vi "PIMAX_1.vi"() -> ()   [LabVIEW 2018]
uses:
  <vilib>/Enthought/Python Integration Toolkit/api/Console Visibility.ctl
  Global Variables.vi
  <vilib>/Enthought/Python Integration Toolkit/Python Integration Toolkit.lvlib
panel:
  in  "Experiment Name":string="TestCamera"
  in  "Logfile?":bool
  in  "File Path":path=path "C:/Labview Test Data/2018-10-09/UnspecifiedProj/Temp Dependence/PIMAX_1_500C_9"
  in  "stop":bool
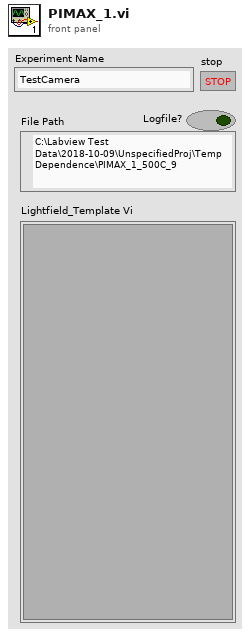
[diagram p1: front panel]
types:
  T1 = typedef "Python Integration Toolkit.lvlib/Console Visibility.ctl" = enum16{"Show Console", "Show Console While Running", "Hide Console"}
  T2 = enum32{"Bad", "Idle", "Run top level", "Running"}
  T3 = typedef "Python Integration Toolkit.lvlib/Session ID.ctl" = u64
  T4 = cluster{"Project":u16, "SubFolder":string, "Filename (Meas. Description)":string, "Measurement index":i32}
  T5 = typedef "Python Integration Toolkit.lvlib/Python Objects.ctl" = variant
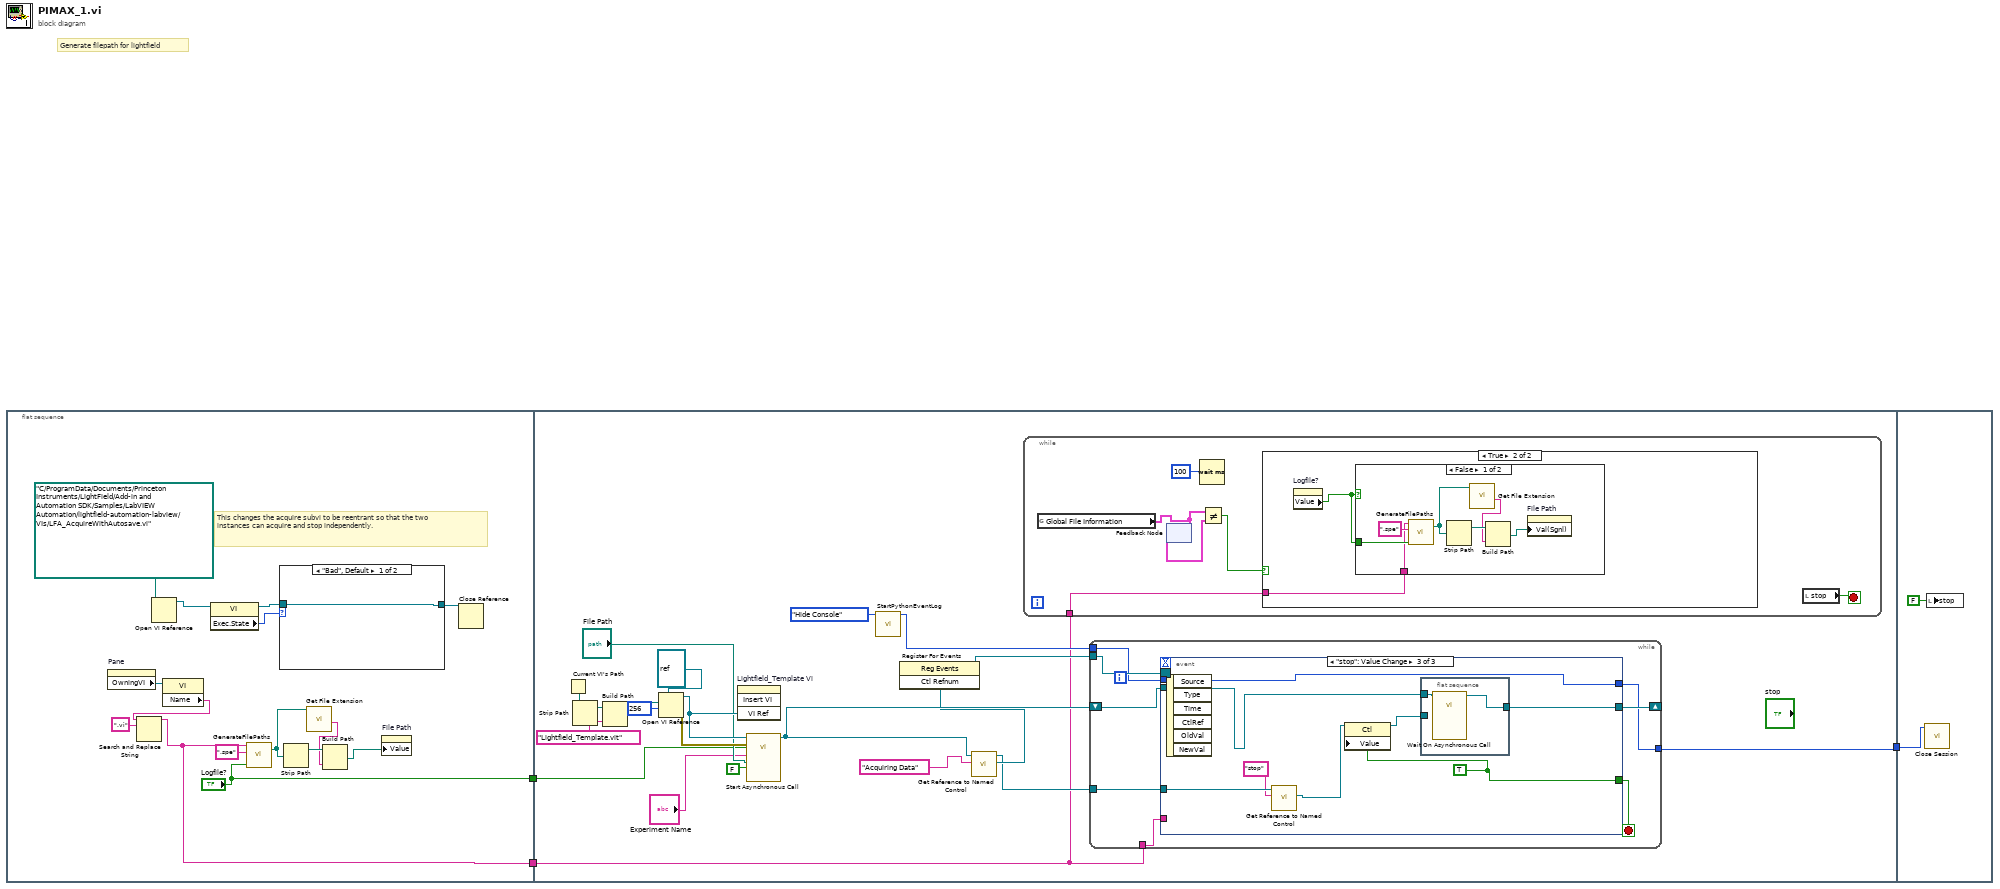
[diagram p0: block diagram]
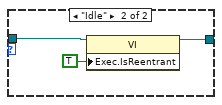
[diagram p2: hidden frame]
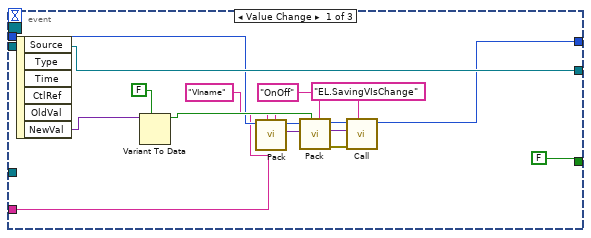
[diagram p5: hidden frame]
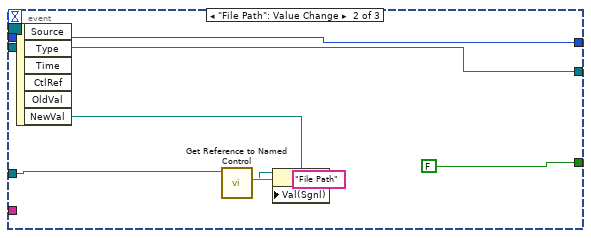
[diagram p6: hidden frame]
diagram:
  # "Generate filepath for lightfield"
  n1 = flat-sequence {
    tunnel: [w5] -> w2
    tunnel: ["Logfile?"] -> w1
    tunnel: [w32] -> w3
    tunnel: w2 -> [w25]
    tunnel: w1 -> [w24]
    tunnel: w3 -> [w100]
    frame #0 {
      # "This changes the acquire subvi to be reentrant so that the two instances can acquire and stop independently."
      n2 = property on="Pane" class="Pane"() -> ("OwningVI"=w8:refnum<vi>)  [unwired: 2 in, 2 out]
      n3 = Open VI Reference(vi path=path "C:/ProgramData/Documents/Princeton Instruments/LightField/Add-in and Automation SDK/Samples/LabVIEW Automation/lightfield-automation-labview/VIs/LFA_AcquireWithAutosave.vi") -> (vi reference=w11:refnum<vi>)  [unwired: 5 in, 1 out]
      n4 = property class="VI"(reference=w8) -> ("Name"=w6:string)  [unwired: 1 in, 2 out]
      n5 = Search and Replace String(input string=w6, search string=".vi") -> (result string=w5:string)  [unwired: 6 in, 3 out]
      n6 = property class="VI"(reference=w11) -> (reference out=w9:refnum<vi>, "Exec.State"=w10:T2)  [unwired: 1 in, 1 out]
      n7 = call "GenerateFilePaths.vi"("Logfile? (F)"="Logfile?", "Extension (.tdms)"=".spe" ("Extension"), "Device Name"=w5) -> ("Path"=w15:path)  [unwired: 2 in]
      n8 = case shown="\"Bad\", Default" w10 {
        tunnel: [w19 w21] -> w17
        tunnel: w9 -> [w19 w20]
        frame "Bad", Default {
        }
        frame "Idle" {
          n9 = property class="VI"(reference=w20, "Exec.IsReentrant"=TRUE ("Execution:Is Reentrant")) -> (reference out=w21:refnum<vi>)  [unwired: 1 in, 1 out]
        }
      }
      n10 = Strip Path(path=w15) -> (stripped path=w14:path)  [unwired: 1 out]
      n11 = call <vilib>:"Get File Extension.vi"("file"=w15) -> ("filename without extension"=w13:string)  [unwired: 6 in, 4 out]
      n12 = Build Path(base path=w14, name or relative path=w13) -> (appended path=w12:path)
      n13 = property on="File Path" class="Path"("Value"=w12) -> ()  [unwired: 2 in, 2 out]
      n14 = Close Reference(reference=w17) -> ()  [unwired: 1 in, 1 out]
    }
    frame #1 {
      n15 = Current VI's Path() -> (path=w42:path)
      n16 = Strip Path(path=w42) -> (stripped path=w43:path)  [unwired: 1 out]
      n17 = Build Path(base path=w43, name or relative path="Lightfield_Template.vit") -> (appended path=w39:path)
      n18 = Open VI Reference(type specifier VI Refnum (for type only)=refnum<vi> refnum, vi path=w39, options=256) -> (vi reference=w38:refnum<vi>, error out=w37:errorcluster)  [unwired: 1 in, 2 out]
      n19 = invoke on="Lightfield_Template Vi" class="SubPnl" method="Insert VI"("VI Ref"=w38) -> ()  [unwired: 3 in, 4 out]
      n20 = call-by-ref "Start Asynchronous Call"(reference=w38, error in=w37, "Add Time to filename"=w24, "Single Run"=FALSE, "File Path"="File Path", "Experiment Name"="Experiment Name") -> (reference out=w31:refnum<vi>)  [unwired: 8 in, 1 out]
      n21 = call "StartPythonEventLog.vi"("Console Visibility"=Console_Visibility."Hide Console") -> ("Session ID out"=w33:T3)  [unwired: 10 in]
      n22 = call "Get Reference to Named Control.vi"("Control Name"="Acquiring Data" ("element"), "Front Panel Ref"=w31) -> ("Ctl Refnum"=w29:refnum<vi>, "Panel Ref Out"=w28:refnum<vi>)  [unwired: 7 in, 1 out]
      n23 = register-events(w29) -> (reference out=w34:refnum<event-registration>)  [unwired: 2 in, 1 out]
      n24 = while {
        tunnel: w25 -> [w44]
        stop <- w49 stop-if-true
        n25 = global read "Global Variables.vi" "Global File Information"() -> (w47:T4)
        n26 = feedback #1() -> (w46:T4)  [unwired: 1 in]
        n27 = feedback-in #1(w47) -> ()
        n28 = Wait (ms)(milliseconds to wait=100) -> ()  [unwired: 1 out]
        n29 = Not Equal?(x=w47, y=w46) -> (x != y?=w45:bool)
        n30 = case shown="True" w45 {
          tunnel: w44 -> [_ w50]
          frame False {
          }
          frame True {
            n31 = property on="Logfile?" class="Bool (strict)"() -> ("Value"=w51:bool)  [unwired: 2 in, 2 out]
            n32 = case shown="False" w51 {
              tunnel: w51 -> [w54 _]
              tunnel: w50 -> [w52 _]
              frame False {
                n33 = call "GenerateFilePaths.vi"("Logfile? (F)"=w54, "Extension (.tdms)"=".spe" ("Extension"), "Device Name"=w52) -> ("Path"=w57:path)  [unwired: 2 in]
                n34 = Strip Path(path=w57) -> (stripped path=w56:path)  [unwired: 1 out]
                n35 = call <vilib>:"Get File Extension.vi"("file"=w57) -> ("filename without extension"=w55:string)  [unwired: 6 in, 4 out]
                n36 = Build Path(base path=w56, name or relative path=w55) -> (appended path=w53:path)
                n37 = property on="File Path" class="Path"("Val(Sgnl)"=w53) -> ()  [unwired: 2 in, 2 out]
              }
              frame True {
              }
            }
          }
        }
        n38 = local read "stop"() -> (w49:bool)
      }
      n39 = while {
        shift-right: [w64] -> _
        shift-left: w31 -> [w65]
        tunnel: w34 -> [w63]
        tunnel: w33 -> [w62]
        tunnel: [w61] -> w32
        tunnel: w28 -> [w60]
        tunnel: w25 -> [w59]
        stop <- w66 stop-if-true
        n40 = event shown="[2] \"stop\": Value Change" {
          selector: w63 -> [_ _ _]
          dyn-events: _ -> [_ _ _]
          timeout: _ -> [_ _ _]
          tunnel: [FALSE FALSE w97] -> w66
          tunnel: w65 -> [w81 w87 w96]
          tunnel: [w81 w87 w95] -> w64
          tunnel: w62 -> [w75 w83 w90]
          tunnel: [w68 w83 w90] -> w61
          tunnel: w60 -> [_ w85 w93]
          tunnel: w59 -> [w67 _ _]
          event Value Change {
            n41 = event-data() -> ("NewVal"=w80:variant)  [unwired: 1 in, 5 out]
            n42 = Variant To Data(type=FALSE, Variant=w80) -> (data=w78:bool)  [unwired: 1 in, 1 out]
            n43 = call <vilib>:"Pack.vi"("Keyword Name"="VIname", "Argument"=w67, "Session ID"=w75) -> ("Python Object References Out"=w70:T5, "Session ID out"=w74:T3)  [unwired: 6 in, 1 out]
            n44 = call <vilib>:"Pack.vi"("Keyword Name"="OnOff", "Argument"=w78, "Python Object References In"=w70, "Session ID"=w74) -> ("error out"=w73:errorcluster, "Python Object References Out"=w72:T5, "Session ID out"=w71:T3)  [unwired: 5 in]
            n45 = call <vilib>:"Call.vi"("Function or Method Name"="EL.SavingVIsChange", "error in (no error)"=w73, "Python Object References In"=w72, "Session ID"=w71) -> ("Session ID out"=w68:T3)  [unwired: 5 in, 2 out]
          }
          event "File Path": Value Change {
            n46 = event-data() -> ("NewVal"=w89:path)  [unwired: 1 in, 5 out]
            n47 = call "Get Reference to Named Control.vi"("Control Name"="File Path" ("element"), "Front Panel Ref"=w85) -> ("Ctl Refnum"=w84:refnum<vi>)  [unwired: 7 in, 2 out]
            n48 = property class="Ctl"(reference=w84, "Val(Sgnl)"=w89) -> ()  [unwired: 1 in, 2 out]
          }
          event "stop": Value Change {
            w97 = TRUE
            n49 = event-data() -> ()  [unwired: 1 in, 6 out]
            n50 = call "Get Reference to Named Control.vi"("Control Name"="stop", "Front Panel Ref"=w93) -> ("Ctl Refnum"=w91:refnum<vi>)  [unwired: 7 in, 2 out]
            n51 = property class="Ctl"(reference=w91, "Value"=w97) -> (reference out=w94:refnum<vi>)  [unwired: 1 in, 1 out]
            n52 = flat-sequence {
              tunnel: w96 -> [w99]
              tunnel: w94 -> [_]
              tunnel: [w98] -> w95
              frame #0 {
                n53 = call-by-ref "Wait On Asynchronous Call"(reference=w99) -> (reference out=w98:refnum<vi>)  [unwired: 13 in, 1 out]
              }
            }
          }
        }
      }
    }
    frame #2 {
      n54 = call <vilib>:"Close Session.vi"("Session ID"=w100) -> ()  [unwired: 10 in, 1 out]
      n55 = local write "stop"(FALSE ("stop")) -> ()
    }
  }
